vi "DAQ_TCP_init.vi"(6 "timeout ms (60000)":i32=60000, 8 "error in":errorcluster, 9 "remote port or service name":u16, 10 "DAQ refDes":string, 11 "address":string) -> (0 "error out":errorcluster, 2 "TCP Success?":bool, 3 "connection ID":refnum<k5>)   [LabVIEW 2024]
panel:
  out "length":i32
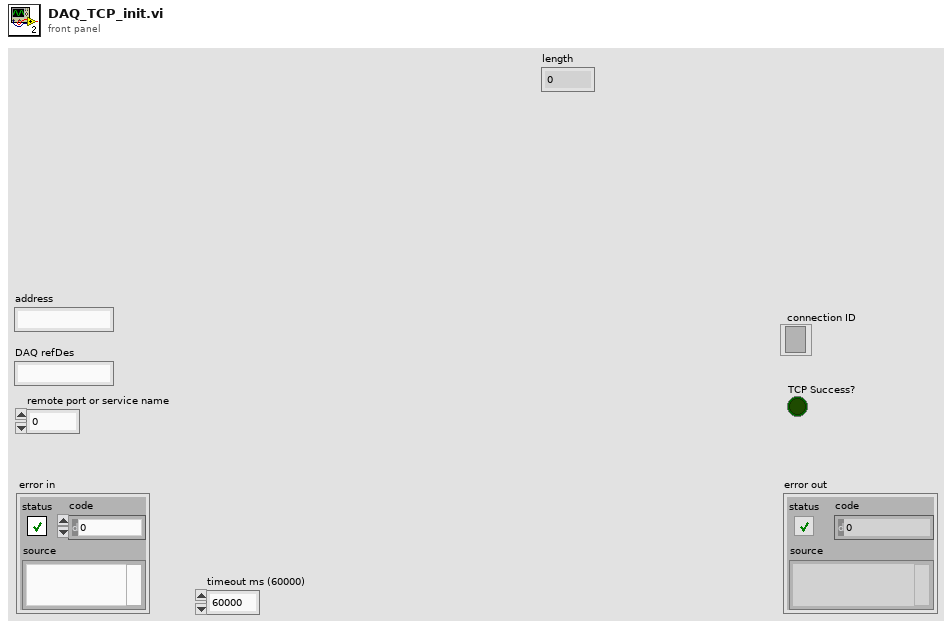
[diagram p1: front panel]
types:
  T1 = enum16{"Standard", "Buffered", "CRLF", "Immediate"}
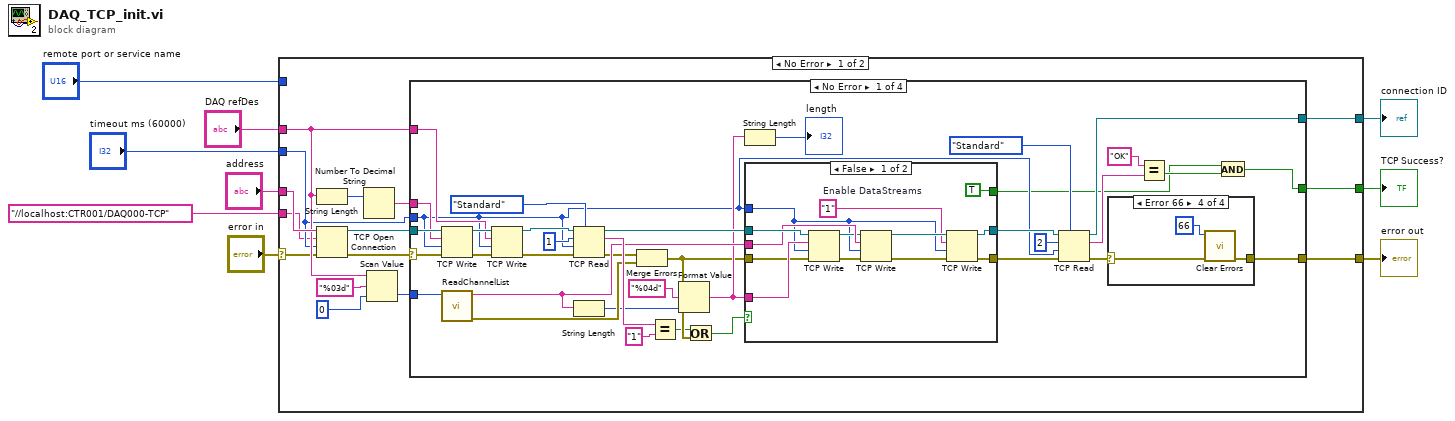
[diagram p0: block diagram]
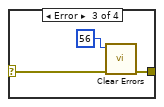
[diagram p4: hidden frame]
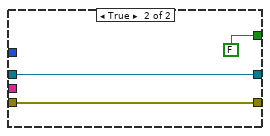
[diagram p5: hidden frame]
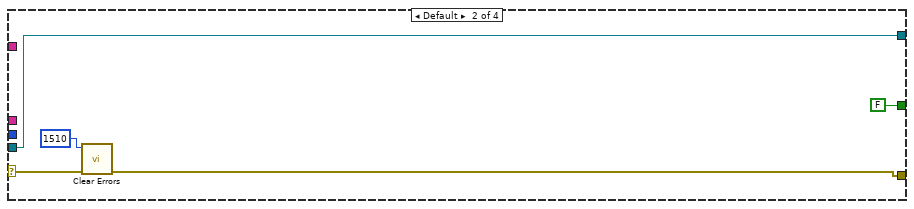
[diagram p6: hidden frame]
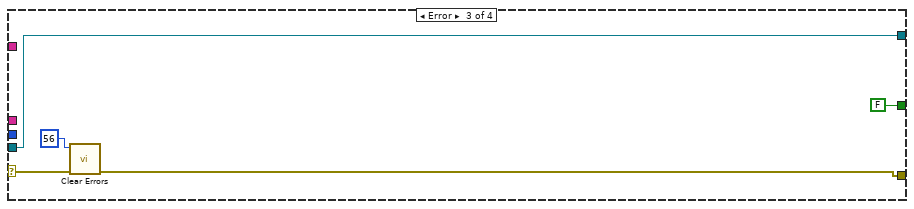
[diagram p7: hidden frame]
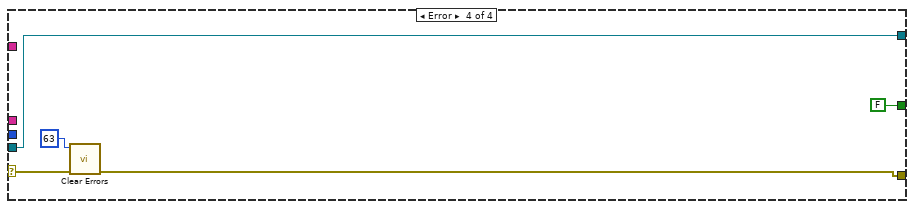
[diagram p8: hidden frame]
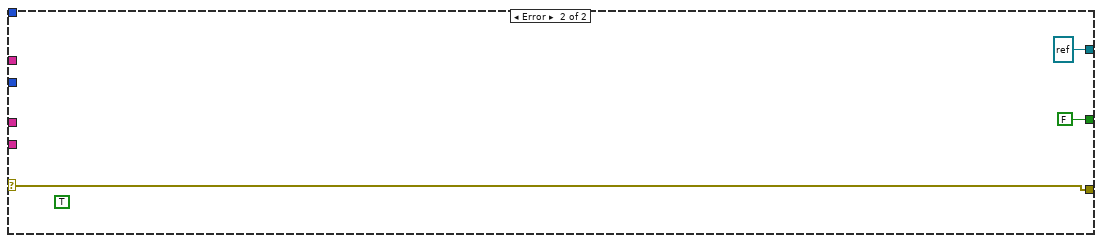
[diagram p9: hidden frame]
diagram:
  n1 = case shown="No Error" "error in" {
    selector: "error in" -> [w14 w101]
    tunnel: "address" -> [w24 _]
    tunnel: "remote port or service name" -> [_ _]
    tunnel: "DAQ refDes" -> [w20 _]
    tunnel: [w16 refnum<k5> refnum ("connection ID")] -> w6
    tunnel: "timeout ms (60000)" -> [w11 _]
    tunnel: [w12 FALSE] -> w3
    tunnel: [w13 w101] -> w1
    tunnel: "//localhost:CTR001/DAQ000-TCP" -> [w10 _]
    frame No Error {
      n2 = String Length(string=w20) -> (length=w23:i32)
      n3 = TCP Open Connection(address=w24, remote port or service name=w10, timeout ms (60000)=w11, error in (no error)=w14) -> (connection ID=w22:refnum<k5>, error out=w15:errorcluster)  [unwired: 1 in]
      n4 = Number To Decimal String(number=w23) -> (decimal integer string=w21:string)  [unwired: 1 in]
      n5 = Scan Value(string=w20, format string="%03d", default (0 dbl)=0) -> (value=w17:i32)  [unwired: 1 out]
      n6 = case shown="No Error" w15 {
        selector: w15 -> [w39 w88 w93 w98]
        tunnel: w22 -> [w60 w89 w94 w99]
        tunnel: w21 -> [w51 _ _ _]
        tunnel: w20 -> [w50 _ _ _]
        tunnel: w17 -> [w49 _ _ _]
        tunnel: [w44 w89 w94 w99] -> w16
        tunnel: w11 -> [w34 _ _ _]
        tunnel: [w25 FALSE FALSE FALSE] -> w12
        tunnel: [w32 w87 w92 w96] -> w13
        frame No Error {
          n7 = TCP Write(connection ID=w60, data in=w51, error in (no error)=w39, 9:w34) -> (connection ID out=w59:refnum<k5>, error out=w61:errorcluster)  [unwired: 1 out]
          n8 = call "ReadChannelList.vi"("DAQ ID #"=w49) -> ("error out"=w52:errorcluster, "Read Channels"=w47:string)  [unwired: 9 in]
          n9 = TCP Write(connection ID=w59, data in=w50, error in (no error)=w61, 9:w34) -> (connection ID out=w58:refnum<k5>, error out=w53:errorcluster)  [unwired: 1 out]
          n10 = TCP Read(connection ID=w58, bytes to read=1, error in (no error)=w53, 7:T1."Standard" ("mode (standard)"), 9:w34) -> (connection ID out=w48:refnum<k5>, data out=w55:string, error out=w31:errorcluster)
          n11 = String Length(string=w47) -> (length=w38:i32)
          n12 = Merge Errors(w31, w52) -> (w29:errorcluster)
          n13 = Equal?(x=w55, y="1") -> (x = y?=w28:bool)
          n14 = Format Value(format string="%04d", value (0)=w38) -> (output string=w36:string)  [unwired: 1 in]
          n15 = Or(x=w28, y=w29) -> (x .or. y?=w30:bool)
          n16 = String Length(string=w36) -> (length=→"length":i32)
          n17 = case shown="False" w30 {
            tunnel: [w74 w84] -> w46
            tunnel: w48 -> [w82 w85]
            tunnel: [w73 w85] -> w45
            tunnel: w36 -> [w81 _]
            tunnel: w34 -> [w72 _]
            tunnel: w47 -> [w79 _]
            tunnel: w29 -> [w71 w84]
            tunnel: [TRUE FALSE] -> w26
            frame False {
              w75 = "1"  # Enable DataStreams
              n18 = TCP Write(connection ID=w82, data in=w81, error in (no error)=w71, 9:w72) -> (connection ID out=w78:refnum<k5>, error out=w80:errorcluster)  [unwired: 1 out]
              n19 = TCP Write(connection ID=w78, data in=w79, error in (no error)=w80, 9:w72) -> (connection ID out=w76:refnum<k5>, error out=w77:errorcluster)  [unwired: 1 out]
              n20 = TCP Write(connection ID=w76, data in=w75, error in (no error)=w77, 9:w72) -> (connection ID out=w73:refnum<k5>, error out=w74:errorcluster)  [unwired: 1 out]
            }
            frame True {
            }
          }
          n21 = TCP Read(connection ID=w45, bytes to read=2, error in (no error)=w46, 7:T1."Standard" ("mode (standard)"), 9:w34) -> (connection ID out=w44:refnum<k5>, data out=w41:string, error out=w33:errorcluster)
          n22 = case shown="Error 66" w33 {
            selector: w33 -> [w62 w63 w65 w68]
            tunnel: [w62 w63 w66 w69] -> w32
            frame No Error {
            }
            frame Default {
            }
            frame Error {
              n23 = call <vilib>:"Clear Errors.vi"("error in (no error)"=w65, "specific error code to clear (0: all)"=56) -> ("error out"=w66:errorcluster)  [unwired: 4 in, 1 out]
            }
            frame Error {
              n24 = call <vilib>:"Clear Errors.vi"("error in (no error)"=w68, "specific error code to clear (0: all)"=66) -> ("error out"=w69:errorcluster)  [unwired: 4 in, 1 out]
            }
          }
          n25 = Equal?(x="OK", y=w41) -> (x = y?=w27:bool)
          n26 = And(x=w26, y=w27) -> (x .and. y?=w25:bool)
        }
        frame Default {
          n27 = call <vilib>:"Clear Errors.vi"("error in (no error)"=w88, "specific error code to clear (0: all)"=1510) -> ("error out"=w87:errorcluster)  [unwired: 4 in, 1 out]
        }
        frame Error {
          n28 = call <vilib>:"Clear Errors.vi"("error in (no error)"=w93, "specific error code to clear (0: all)"=56) -> ("error out"=w92:errorcluster)  [unwired: 4 in, 1 out]
        }
        frame Error {
          n29 = call <vilib>:"Clear Errors.vi"("error in (no error)"=w98, "specific error code to clear (0: all)"=63) -> ("error out"=w96:errorcluster)  [unwired: 4 in, 1 out]
        }
      }
    }
    frame Error {
      (unwired) TRUE
    }
  }
  "error out" <- w1
  "connection ID" <- w6
  "TCP Success?" <- w3
